vi "Camera Toggle.vi"(11 "Toggle In":bool) -> (0 "Current Cam":string)   [LabVIEW 2018]
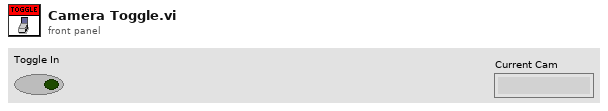
[diagram p1: front panel]
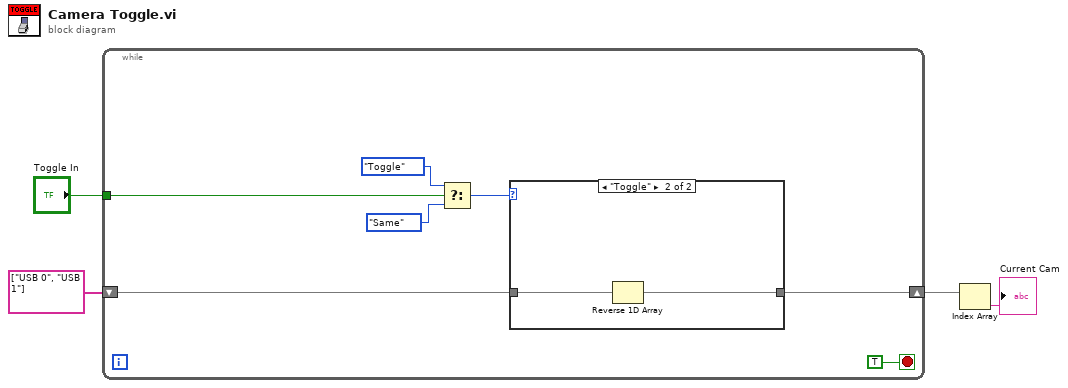
[diagram p0: block diagram]
diagram:
  n1 = while {
    shift-right: [w6] -> w3
    shift-left: string[] ["USB 0", "USB 1"] -> [w7]
    tunnel: "Toggle In" -> [w5]
    stop <- TRUE stop-if-true
    n2 = Select(t=enum16{"Same", "Toggle"}."Toggle", s=w5, f=enum16{"Same", "Toggle"}."Same") -> (s? t:f=w8:enum16{"Same", "Toggle"})
    n3 = case shown="\"Toggle\"" w8 {
      tunnel: w7 -> [w12 w14]
      tunnel: [w12 w13] -> w6
      frame "Same", Default {
      }
      frame "Toggle" {
        n4 = Reverse 1D Array(array=w14) -> (reversed array=w13:string[])
      }
    }
  }
  n5 = Index Array(array=w3) -> (element=→"Current Cam":string)  [unwired: 1 in]
